vi "robotic module.vi"(10 "Repeat (MUST BE 1)":i32, 11 "motion type":i64) -> (3 "array":i32[][](array[numeric]))   [LabVIEW 2019]
doc: "For setting robotic arm position"
uses:
  <vilib>/imath/engines/lvmath2/RunTimeEngine/Managers/WorkSpace/UID Generator.vi
  <vilib>/imath/engines/lvmath2/RunTimeEngine/IndexRead/NIMS V(S).vi
  <instcachedir>/0/NIMS V(S)_0488751826AF41519A22953C041130DC.lvgen/NIMS V(S)_0488751826AF41519A22953C041130DC_002.vi
  <vilib>/imathl/engines/lvmath/Functions/Error Handling/Create Error.vi
  <vilib>/imath/engines/lvmath2/RunTimeEngine/ErrorHandling/NIMS_Create Error From Enums.vi
  <vilib>/imath/engines/lvmath2/RunTimeEngine/RunTimeType/NIMS_RunTimeType_From StrictType (excl LVString).vi
  <instcachedir>/0/NIMS_RunTimeType_From StrictType (excl LVString)_D8AFBA86A94845AAA577C895450664BD.lvgen/NIMS_RunTimeType_From StrictType (excl LVString)_D8AFBA86A94845AAA577C895450664BD_000.vi
  <vilib>/imath/engines/lvmath2/RunTimeEngine/LocalVariableDefStatement/MC_LocalVariableDefStatement_Display.vi
  <vilib>/imath/engines/lvmath2/RunTimeEngine/Managers/SymbolTable/Clear UID.vi
  <vilib>/imath/engines/lvmath2/RunTimeEngine/NodeEndStatement/NIMS_NodeEndStatement_Output.vi
  <instcachedir>/0/NIMS_NodeEndStatement_Output_53EC0D466D134D7ABD903AC30B43404B.lvgen/NIMS_NodeEndStatement_Output_53EC0D466D134D7ABD903AC30B43404B_010.vi
  <instcachedir>/0/NIMS_NodeEndStatement_Output_53EC0D466D134D7ABD903AC30B43404B.lvgen/NIMS_NodeEndStatement_Output_53EC0D466D134D7ABD903AC30B43404B_011.vi
  <vilib>/imath/engines/lvmath2/RunTimeEngine/ErrorHandling/NIMS_Finalize Error.vi
  <vilib>/imath/engines/lvmath2/RunTimeEngine/Managers/SymbolTable/NIMS_WorkSpace.lvlib
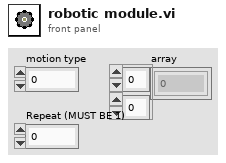
[diagram p1: front panel]
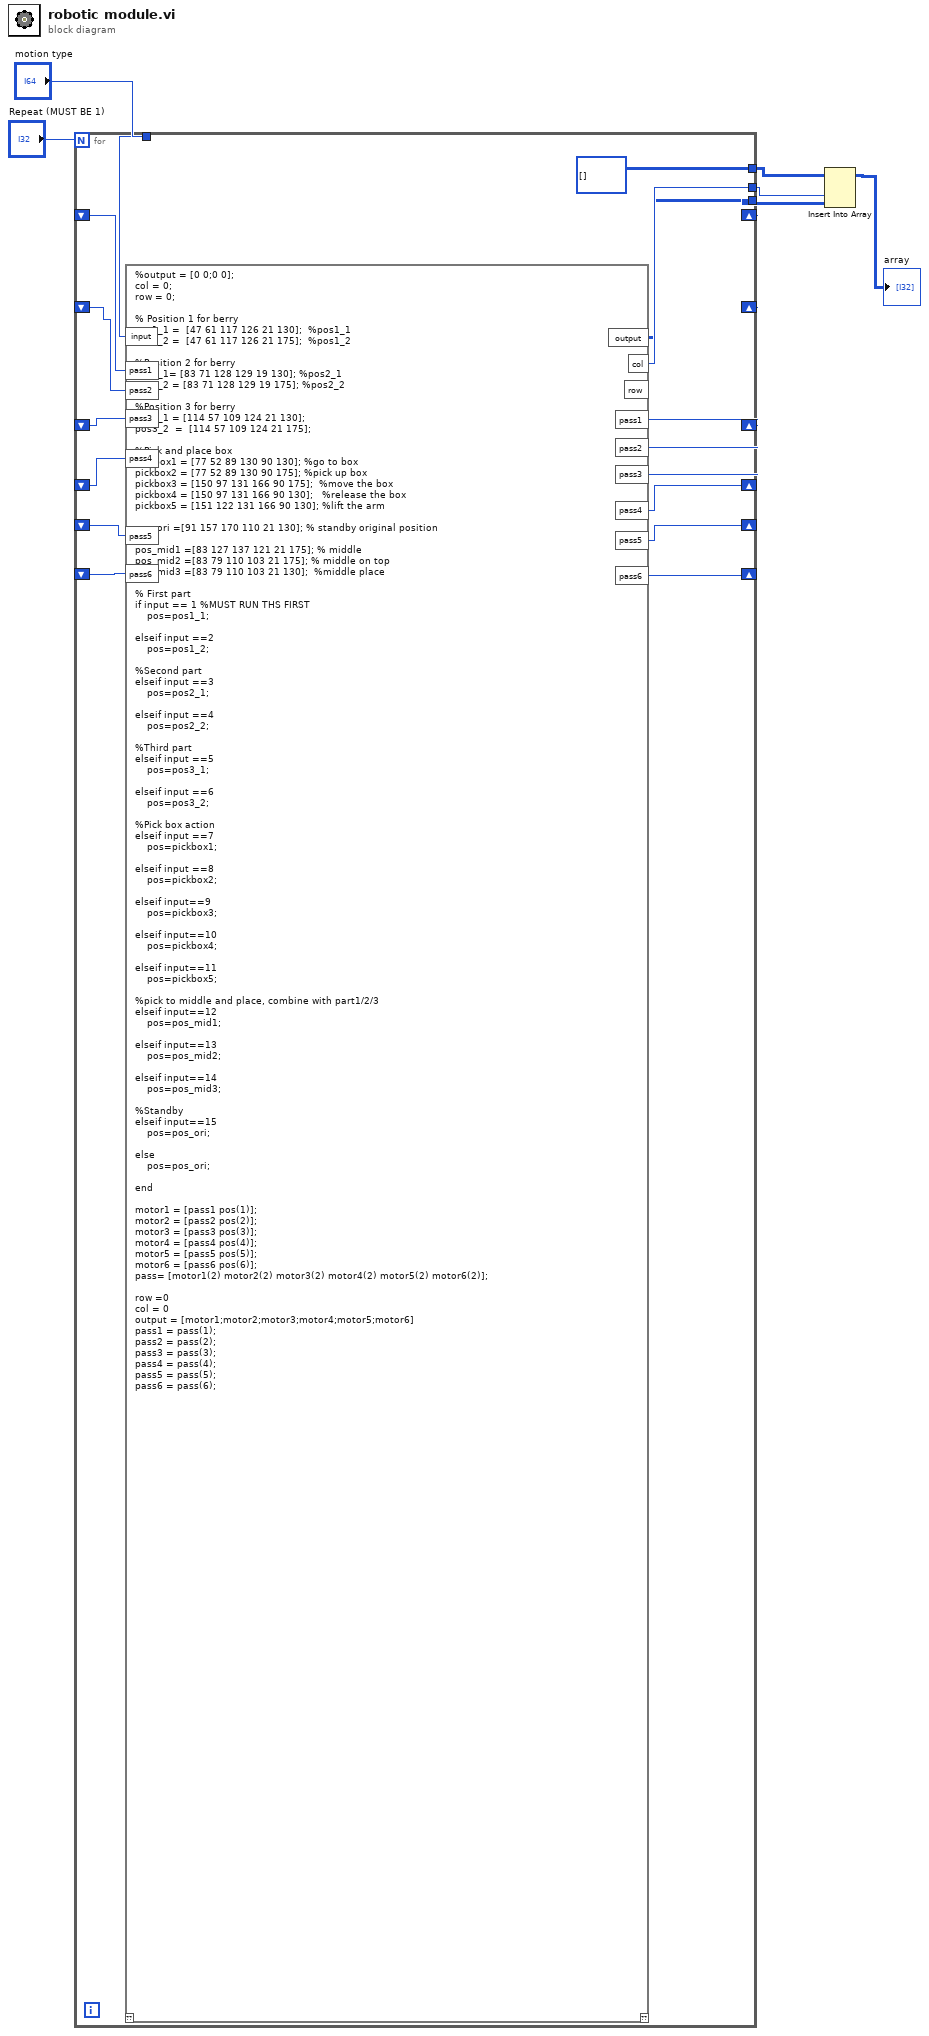
[diagram p0: block diagram]
diagram:
  n1 = for {
    N: "Repeat (MUST BE 1)" -> [_]
    tunnel: "motion type" -> [w22]
    shift-right: [w21] -> _
    shift-left: _ -> [w20]
    shift-right: [w19] -> _
    shift-left: _ -> [w18]
    shift-right: [w17] -> _
    shift-left: _ -> [w16]
    shift-right: [w14] -> _
    shift-left: _ -> [w15]
    tunnel: [i32[][] [] ("array")] -> w3
    tunnel: [w12] -> w4
    tunnel: [w11] -> w5
    shift-right: [w9] -> _
    shift-left: _ -> [w10]
    shift-right: [w7] -> _
    shift-left: _ -> [w8]
    n2 = mathscript code="%output = [0 0;0 0];\ncol = 0;\nrow = 0;\n\n% Position 1 for berry\npos1_1 =  [47 61 117 126 21 130];  %pos1_1\npos1_2 =  [47 61 117 126 21 175];  %pos1_2\n\n%Position 2 for berry\npos2_1= [83 71 128 129 19 130]; %pos2_1\npos2_2 = [83 71 128 129 19 175]; %pos2_2\n\n%Position 3 for berry\npos3_1 = [114 57 109 124 21 130];\npos3_2  =  [114 57 109 124 21 175];\n\n%Pick and place box\npickbox1 = [77 52 89 130 90 130]; %go to box\npickbox2 = [77 52 89 130 90 175]; %pick up box\npickbox3 = [150 97 131 166 90 175];  %move the box\npickbox4 = [150 97 131 166 90 130];   %release the box\npickbox5 = [151 122 131 166 90 130]; %lift the arm\n\npos_ori =[91 157 170 110 21 130]; % standby original position\n\npos_mid1 =[83 127 137 121 21 175]; % middle \npos_mid2 =[83 79 110 103 21 175]; % middle on top\npos_mid3 =[83 79 110 103 21 130];  %middle place\n\n% First part\nif input == 1 %MUST RUN THS FIRST\n    pos=pos1_1;\n\nelseif input ==2\n    pos=pos1_2;\n\n%Second part\nelseif input ==3\n    pos=pos2_1;\n\nelseif input ==4\n    pos=pos2_2;\n\n%Third part\nelseif input ==5\n    pos=pos3_1;\n\nelseif input ==6\n    pos=pos3_2;\n\n%Pick box action\nelseif input ==7\n    pos=pickbox1;\n\nelseif input ==8\n    pos=pickbox2;\n\nelseif input==9\n    pos=pickbox3;\n\nelseif input==10\n    pos=pickbox4;\n\nelseif input==11\n    pos=pickbox5;\n\n%pick to middle and place, combine with part1/2/3\nelseif input==12\n    pos=pos_mid1;\n\nelseif input==13\n    pos=pos_mid2;\n\nelseif input==14\n    pos=pos_mid3;\n\n%Standby\nelseif input==15\n    pos=pos_ori;\n\nelse\n    pos=pos_ori;\n\nend\n\nmotor1 = [pass1 pos(1)];\nmotor2 = [pass2 pos(2)];\nmotor3 = [pass3 pos(3)];\nmotor4 = [pass4 pos(4)];\nmotor5 = [pass5 pos(5)];\nmotor6 = [pass6 pos(6)];\npass= [motor1(2) motor2(2) motor3(2) motor4(2) motor5(2) motor6(2)];\n\nrow =0\ncol = 0\noutput = [motor1;motor2;motor3;motor4;motor5;motor6]\npass1 = pass(1);\npass2 = pass(2);\npass3 = pass(3);\npass4 = pass(4);\npass5 = pass(5);\npass6 = pass(6);"("input"=w22, "pass1"=w20, "pass2"=w18, "pass3"=w16, "pass4"=w15, "pass5"=w10, "pass6"=w8) -> ("output"=w11:i32[][], "col"=w12:i32, "pass1"=w21:i32, "pass2"=w19:i32, "pass3"=w17:i32, "pass4"=w14:i32, "pass5"=w9:i32, "pass6"=w7:i32)  [unwired: 1 in, 2 out]
  }
  n3 = Insert Into Array(array=w3, index (col)=w4, new element=w5) -> (→"array":i32[][])  [unwired: 1 in]
